vi "Untitled 1.vi"() -> ()   [LabVIEW 2016]
panel:
  out "s3":string
  in  "s1":string
  in  "Stop Button":bool
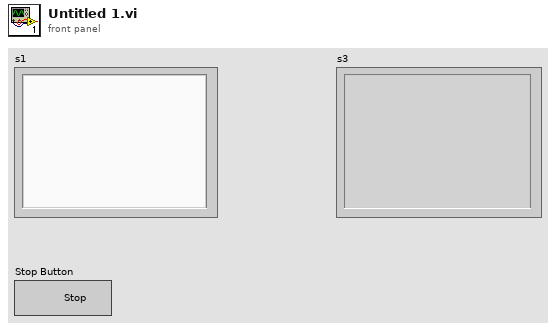
[diagram p1: front panel]
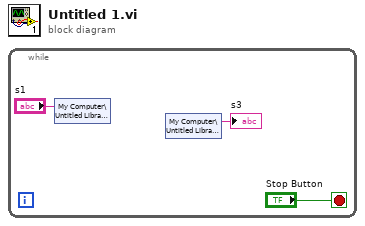
[diagram p0: block diagram]
diagram:
  n1 = while {
    stop <- "Stop Button" stop-if-true
    n2 = shared-variable "My Computer\\Untitled Library 1.lvlib\\s1"("s1") -> ()  [unwired: 1 in, 1 out]
    n3 = shared-variable "My Computer\\Untitled Library 1.lvlib\\s3"() -> (→"s3":string)  [unwired: 1 in, 1 out]
  }
